vi "Translate Data to Virtual Device.vi"() -> ()   [LabVIEW 2015, in "AE75TX Actor.lvlib" / "AE75TX.lvclass"]
uses:
  AE75TX.lvclass
  Controls/PV Full Data Cluster.ctl
  Controls/PV Standard Value Cluster.ctl
panel:
  out "Length":u16
  out "Address":u16
  out "Data Array":u16[](array[numeric])
  out "error out":errorcluster
  in  "error in (no error)":errorcluster
  in  "PV Data":T1
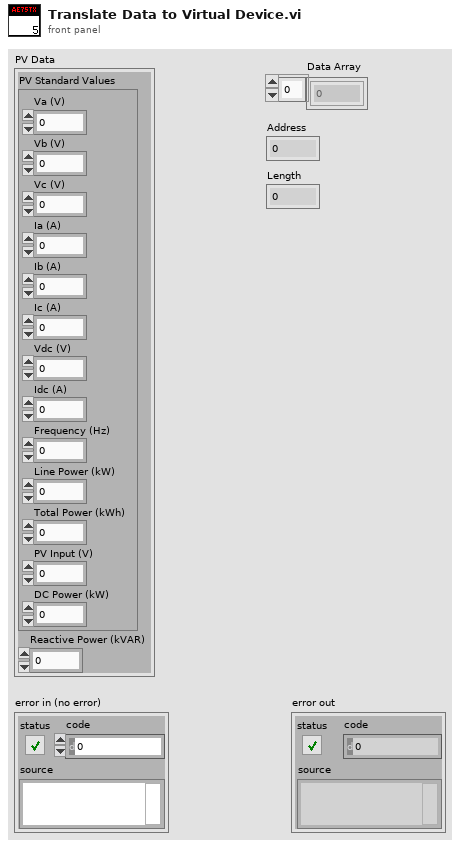
[diagram p1: front panel]
types:
  T1 = typedef "AE75TX Actor.lvlib/AE75TX.lvclass/PV Full Data Cluster.ctl" = cluster{"PV Standard Values":T2, "Reactive Power (kVAR)":sgl}
  T2 = typedef "AE75TX Actor.lvlib/AE75TX.lvclass/PV Standard Value Cluster.ctl" = cluster{"Va (V)":sgl, "Vb (V)":sgl, "Vc (V)":sgl, "Ia (A)":sgl, "Ib (A)":sgl, "Ic (A)":sgl, "Vdc (V)":sgl, "Idc (A)":sgl, "Frequency (Hz)":sgl, "Line Power (kW)":sgl, "Total Power (kWh)":u32, "PV Input (V)":sgl, "DC Power (kW)":sgl}
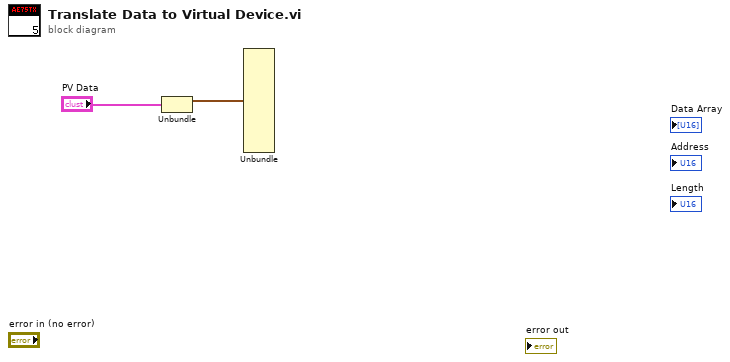
[diagram p0: block diagram]
diagram:
  n1 = Unbundle("PV Data") -> ("PV Standard Values"=w1:T2)  [unwired: 1 out]
  n2 = Unbundle(w1) -> ()  [unwired: 13 out]
